vi "PRBSgenerator.vi"(6 "Action":T2, 8 "error in (no error)":errorcluster, 11 "PRBS Parameters":T1 {"polynomial order" max=512}) -> (0 "error out":errorcluster, 2 "PRBS out":fxp<+/-,20,5>[](array[numeric]), 3 "Finalizado?":bool)   [LabVIEW 2017]
uses:
  PRBScontrol.ctl
  PRBSparameters.ctl
  Setpoints.ctl
  <vilib>/addons/System Identification/NI_SysID.lvlib
panel:
  out "PRBS":u8[][](array[numeric])
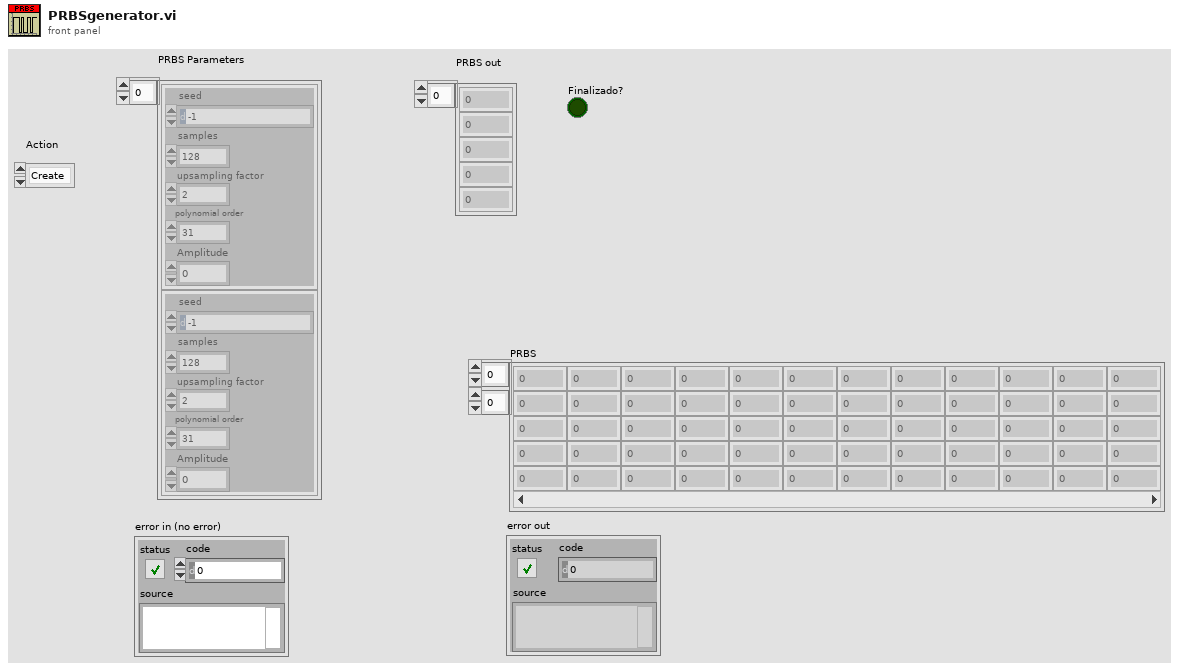
[diagram p1: front panel]
types:
  T1 = typedef "PRBSparameters.ctl" = cluster{"seed":i64, "samples":i64, "upsampling factor":i32, "polynomial order":i32, "Amplitude":dbl}[]
  T2 = typedef "PRBScontrol.ctl" = enum16{"Create", "Get data point"}
  T3 = cluster{"seed":i64, "samples":i64, "upsampling factor":i32, "polynomial order":i32, "Amplitude":dbl}
  T4 = typedef "Setpoints.ctl" = cluster{"Bomba 1":fxp<+/-,20,5>, "Bomba 2":fxp<+/-,20,5>, "Solenoide 1":bool, "Solenoide 2":bool, "Solenoide 3":bool, "Solenoide 4":bool, "Valvula proporcional 2":fxp<+/-,20,5>, "Valvula proporcional 1":fxp<+/-,20,5>}
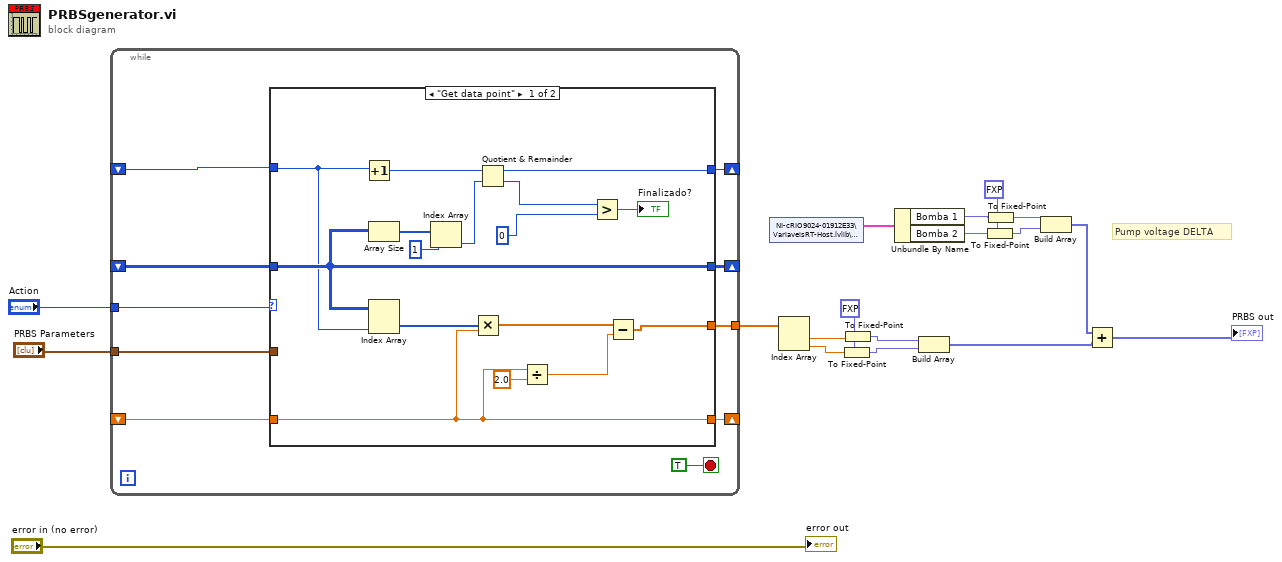
[diagram p0: block diagram]
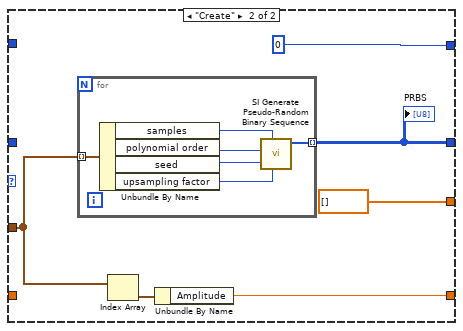
[diagram p2: hidden frame]
diagram:
  w6 = fxp<+/-,19,5> 0.0 ("fixed-point type")
  w15 = fxp<+/-,19,5> 0.0 ("fixed-point type")
  # "Pump voltage DELTA"
  n1 = while {
    tunnel: "Action" -> [w27]
    shift-right: [w26] -> _
    shift-left: _ -> [w25]
    shift-right: [w23] -> _
    shift-left: _ -> [w24]
    tunnel: [w22] -> w16
    tunnel: "PRBS Parameters" -> [w21]
    shift-right: [w20] -> _
    shift-left: _ -> [w19]
    stop <- TRUE stop-if-true
    n2 = case shown="\"Get data point\"" w27 {
      tunnel: [w43 w49] -> w26
      tunnel: w25 -> [w43 _]
      tunnel: w24 -> [w38 _]
      tunnel: [w42 0] -> w23
      tunnel: [w29 dbl[] []] -> w22
      tunnel: w21 -> [_ w47]
      tunnel: [w33 w45] -> w20
      tunnel: w19 -> [w33 _]
      frame "Get data point" {
        n3 = Increment(x=w38) -> (x+1=w44:i32)
        n4 = Array Size(array=w43) -> (size(s)=w41:i32[])
        n5 = Index Array(array=w43, index (col)=w38) -> (element=w34:u8[])  [unwired: 1 in]
        n6 = Index Array(array=w41, index=1) -> (element=w39:i32)
        n7 = Multiply(x=w34, y=w33) -> (x*y=w31:dbl[])
        n8 = Quotient & Remainder(x=w44, y=w39) -> (x-y*floor(x/y)=w42:i32, floor(x/y)=w37:i32)
        n9 = Divide(x=w33, y=2.0) -> (x/y=w30:dbl)
        n10 = Greater?(x=w37, y=0) -> (0:→"Finalizado?":bool)
        n11 = Subtract(x=w31, y=w30) -> (x-y=w29:dbl[])
      }
      frame "Create" {
        n12 = for {
          tunnel: [w52] -> w49 mode=indexing
          tunnel: w47 -> [w51] mode=indexing
          n13 = Unbundle By Name(w51) -> ("samples"=w56:i64, "polynomial order"=w55:i32, "seed"=w54:i64, "upsampling factor"=w53:i32)
          n14 = call <vilib>:"SI Generate Pseudo-Random Binary Sequence.vi"("upsampling factor"=w53, "seed"=w54, "polynomial order"=w55, "samples"=w56) -> ("PRBS"=w52:u8[])  [unwired: 7 in]
        }
        "PRBS" <- w49
        n15 = Index Array(array=w47) -> (element=w46:T3)  [unwired: 1 in]
        n16 = Unbundle By Name(w46) -> ("Amplitude"=w45:dbl)
      }
    }
  }
  n17 = shared-variable "NI-cRIO9024-01912E33\\VariaveisRT-Host.lvlib\\Setpoints"() -> (w17:T4)  [unwired: 1 in, 1 out]
  n18 = Index Array(array=w16) -> (element #1=w14:dbl, element #2=w13:dbl)  [unwired: 2 in]
  n19 = To Fixed-Point(fixed-point type=w15, number=w13) -> (fixed-point=w11:fxp<+/-,19,5>)
  n20 = To Fixed-Point(fixed-point type=w15, number=w14) -> (fixed-point=w12:fxp<+/-,19,5>)
  n21 = Unbundle By Name(w17) -> ("Bomba 1"=w9:fxp<+/-,20,5>, "Bomba 2"=w8:fxp<+/-,20,5>)
  n22 = Build Array(w12, w11) -> (w4:fxp<+/-,19,5>[])
  n23 = To Fixed-Point(fixed-point type=w6, number=w8) -> (fixed-point=w7:fxp<+/-,19,5>)
  n24 = To Fixed-Point(fixed-point type=w6, number=w9) -> (fixed-point=w5:fxp<+/-,19,5>)
  n25 = Build Array(w5, w7) -> (w3:fxp<+/-,19,5>[])
  n26 = Add(x=w3, y=w4) -> (x+y=→"PRBS out":fxp<+/-,20,6>[])
  "error out" <- "error in (no error)"
